vi "GenericGpibDriver.vi"(5 "VISA resource name":refnum<visa-resource-name>, 6 "Command":string) -> (0 "Error Code":i32, 1 "Error Status":bool, 2 "Error source":string, 3 "Bytes Read":dbl, 4 "Return Value":string)   [LabVIEW 2014]
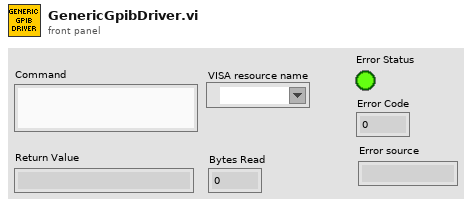
[diagram p1: front panel]
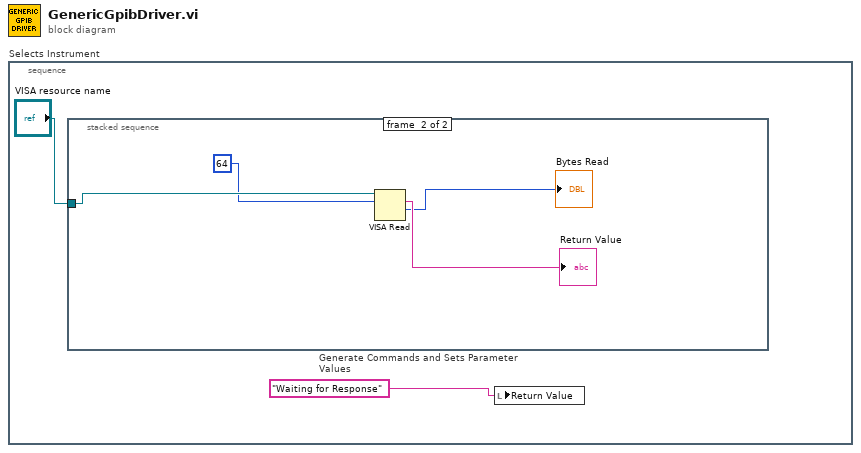
[diagram p0: block diagram]
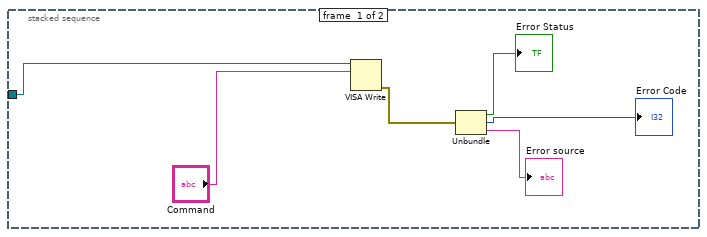
[diagram p2: hidden frame]
diagram:
  n1 = stacked-sequence "Selects Instrument" {
    frame #0 {
      n2 = stacked-sequence "Generate Commands and Sets Parameter Values" {
        tunnel: "VISA resource name" -> [w8 w12]
        frame #0 {
          n3 = VISA Write(VISA resource name=w8, write buffer="Command") -> (error out=w6:errorcluster)  [unwired: 1 in, 2 out]
          n4 = Unbundle(w6) -> ("status"=→"Error Status":bool, "code"=→"Error Code":i32, "source"=→"Error source":string)
        }
        frame #1 {
          n5 = VISA Read(VISA resource name=w12, byte count=64) -> (read buffer=→"Return Value":string, return count=→"Bytes Read":u32)  [unwired: 1 in, 2 out]
        }
      }
      n6 = local write "Return Value"("Waiting for Response") -> ()
    }
  }
